vi "array IO.vi"() -> ()   [LabVIEW 2026]
uses:
  <vilib>/eio/EIONode/EIONode.xnode
  <vilib>/rvi/eio/common/nirviEmuTemplateMethod_errors.vi
panel:
  in  "I/O Item":bool[](array[boolean])=[FALSE, FALSE, FALSE, FALSE]
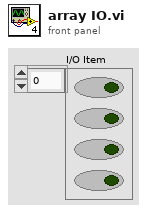
[diagram p1: front panel]
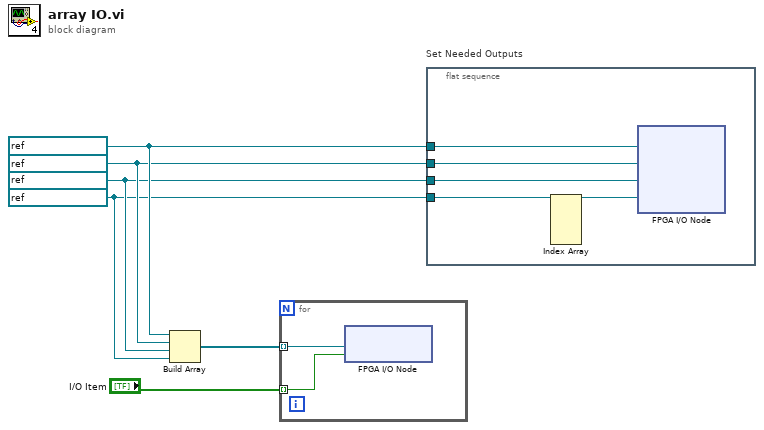
[diagram p0: block diagram]
diagram:
  w3 = refnum<k21> "Bank-03/DO3" ("FPGA I/O In")
  w4 = refnum<k21> "Bank-03/DO2" ("FPGA I/O In")
  w5 = refnum<k21> "Bank-03/DO1" ("FPGA I/O In")
  w6 = refnum<k21> "Bank-03/DO0" ("FPGA I/O In")
  n1 = Build Array(w6, w5, w4, w3) -> (w2:refnum<k21>[])
  n2 = for {
    tunnel: w2 -> [w8] mode=indexing
    tunnel: "I/O Item" -> [w7] mode=indexing
    n3 = xnode "FPGA I/O Node"("I/O Item"=w7, "FPGA I/O In"=w8) -> ()  [unwired: 1 out]
  }
  n4 = flat-sequence "Set Needed Outputs" {
    tunnel: w3 -> [w9]
    tunnel: w4 -> [w12]
    tunnel: w5 -> [w11]
    tunnel: w6 -> [w10]
    frame #0 {
      n5 = Index Array() -> ()  [unwired: 5 in, 4 out]
      n6 = xnode "FPGA I/O Node"("FPGA I/O In"=w10, "FPGA I/O In"=w11, "FPGA I/O In"=w12, "FPGA I/O In"=w9) -> ()  [unwired: 4 in, 4 out]
    }
  }
